vi "main.vi"() -> ()   [LabVIEW 2023, in "task_1.lvlib"]
doc: "A data monitoring system to to acquire and plot data."
uses:
  task_1.lvlib
  Controls/event_operations.ctl
  Controls/data_limits.ctl
  Controls/Queue_op.ctl
  <vilib>/Analysis/Matrix/Numeric/Conversions/Array To Matrix - RA.vi
  <vilib>/Analysis/Matrix/NI_Matrix.lvlib
panel:
  out "LED":bool
  out "error out":errorcluster
  in  "error in (no error)":errorcluster
  out "Temperature (°C):":dbl format="%#_4g"
  out "Current (mA):":dbl format="%#_4g"
  in  "Log Rate":dbl=1.0 min=1.0 step=1.0
  in  "Current. Low Limit mA":dbl min=0.0 max=100.0 format="%#.2g"
  in  "Current. High Limit mA":dbl=100.0 min=0.0 max=100.0 format="%#.2g"
  in  "Temp. Low Limit   °C":dbl min=0.0 max=100.0 format="%#.2g"
  in  "Temp. High Limit °C":dbl=100.0 min=0.0 max=100.0 format="%#.2g"
  in  "Exit":bool
  out "Chart":dbl[][](graph)=[[75.40776627883477, 3.2055013029279156]]
  in  "Start":bool
  # "Data Monitoring System"
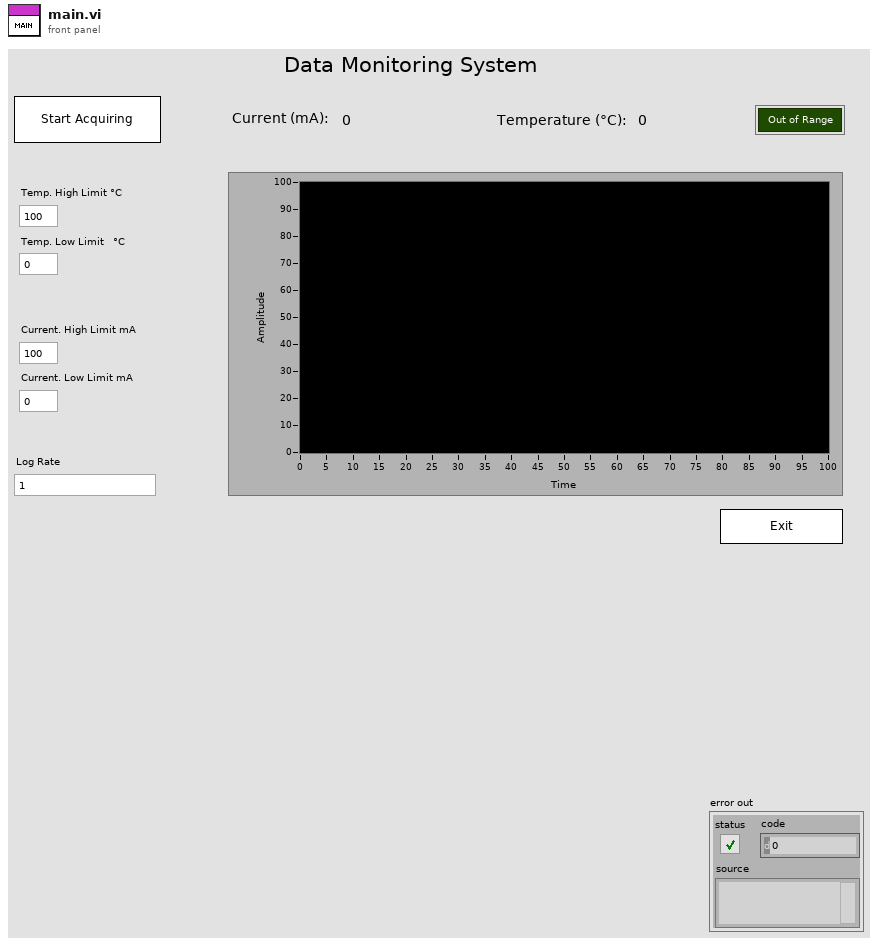
[diagram p1: front panel]
types:
  T1 = typedef "task_1.lvlib/data_limits.ctl" = cluster{"curr_h":dbl, "curr_l":dbl, "temp_h":dbl, "temp_l":dbl, "Acquiring?":bool}
  T2 = typedef "task_1.lvlib/event_operations.ctl" = enum16{"Create", "Generate", "Get_ref", "Destroy"}
  T3 = typedef "task_1.lvlib/Queue_op.ctl" = enum16{"Create", "Enqueue", "Dequeue", "Destroy"}
  T4 = enum32{"Invalid", "Standard", "Closed", "Hidden", "Minimized", "Maximized"}
  T5 = typedef "task_1.lvlib/Data_TC.ctl" = cluster{"Current":dbl, "Temperature":dbl}
  T6 = typedef "NI_Matrix.lvlib/RealMatrix.ctl" = dbl[][]
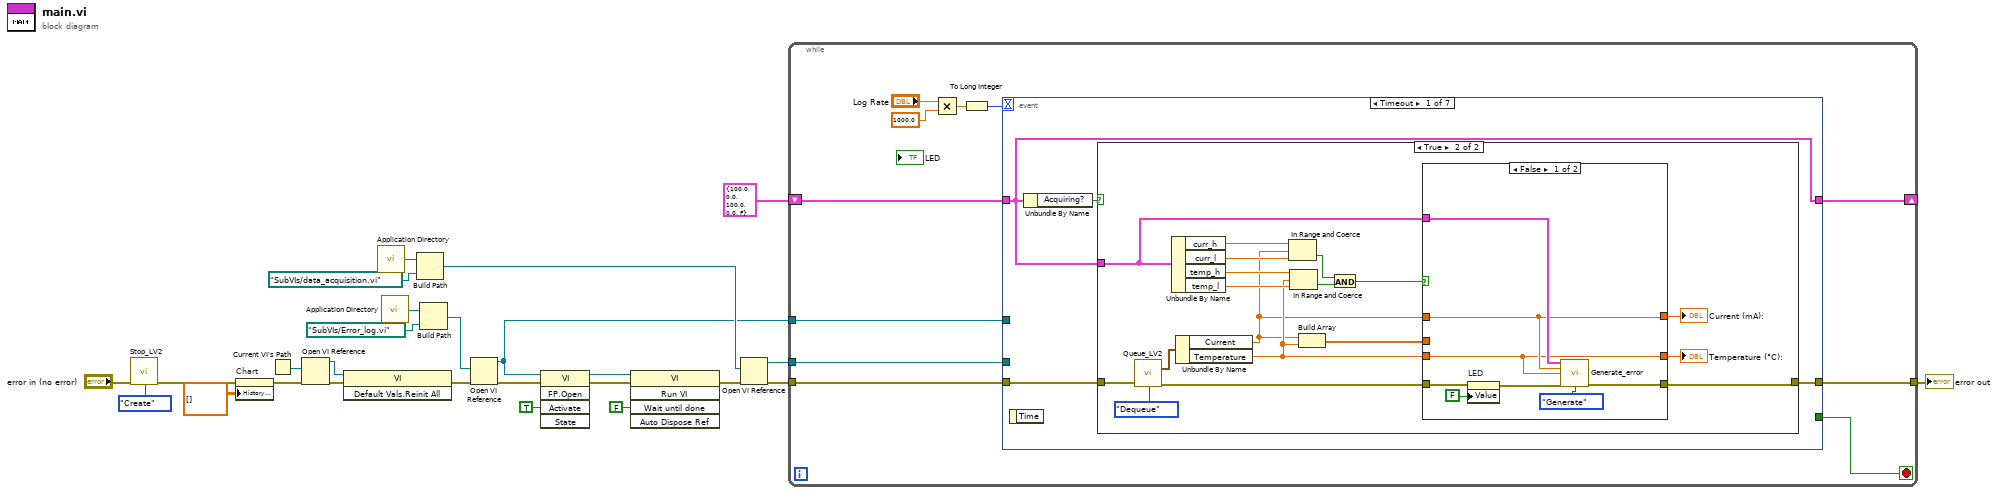
[diagram p0: block diagram]
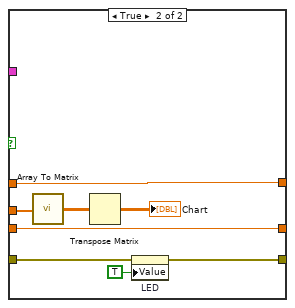
[diagram p3: hidden frame]
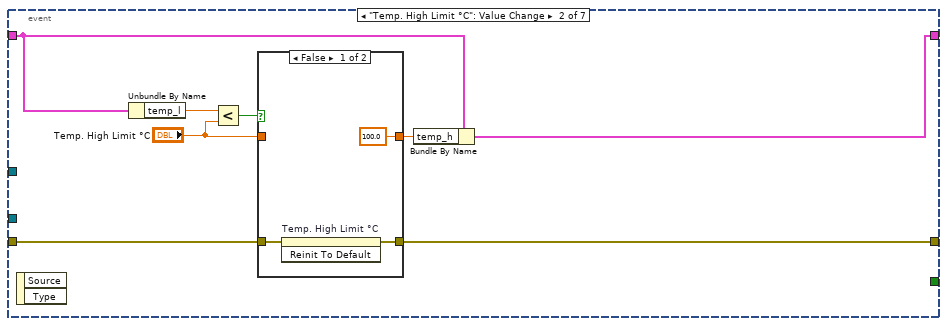
[diagram p4: hidden frame]
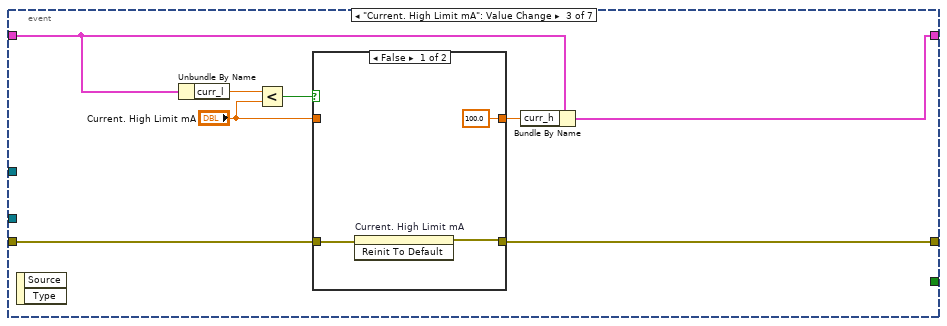
[diagram p6: hidden frame]
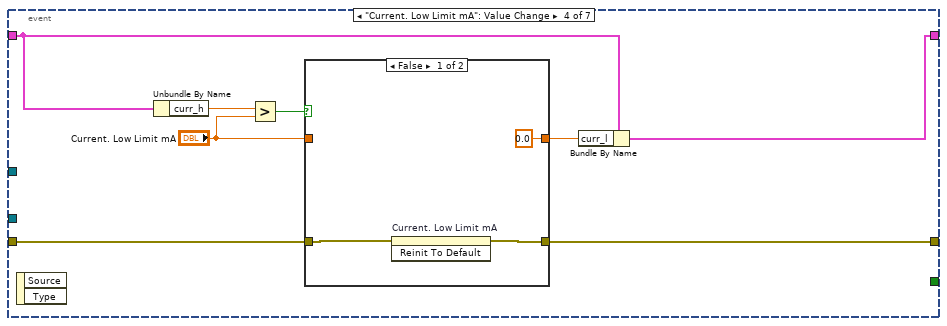
[diagram p8: hidden frame]
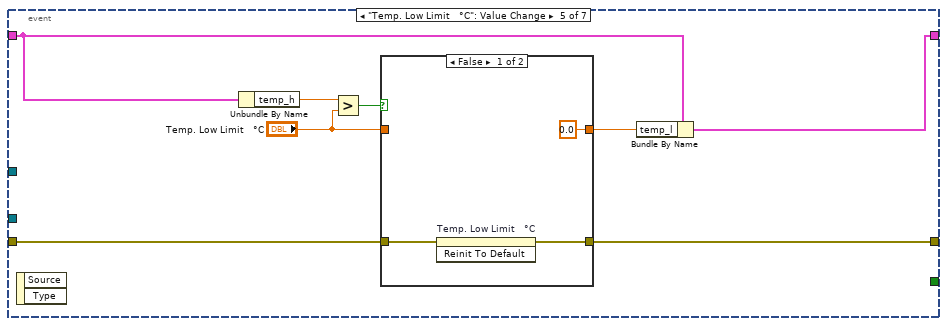
[diagram p10: hidden frame]
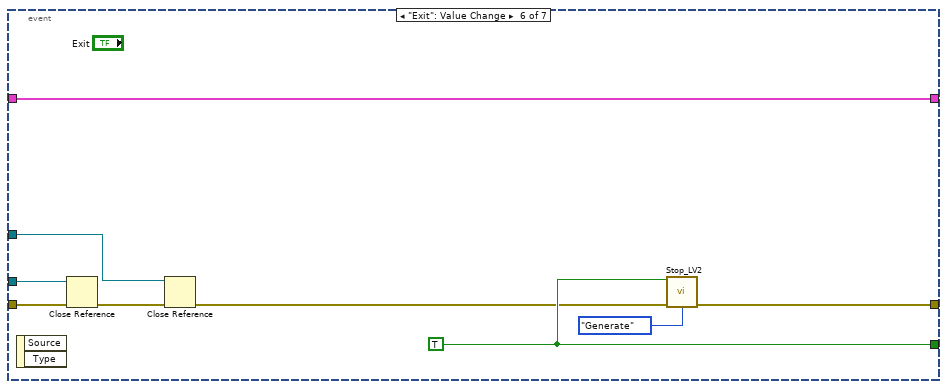
[diagram p12: hidden frame]
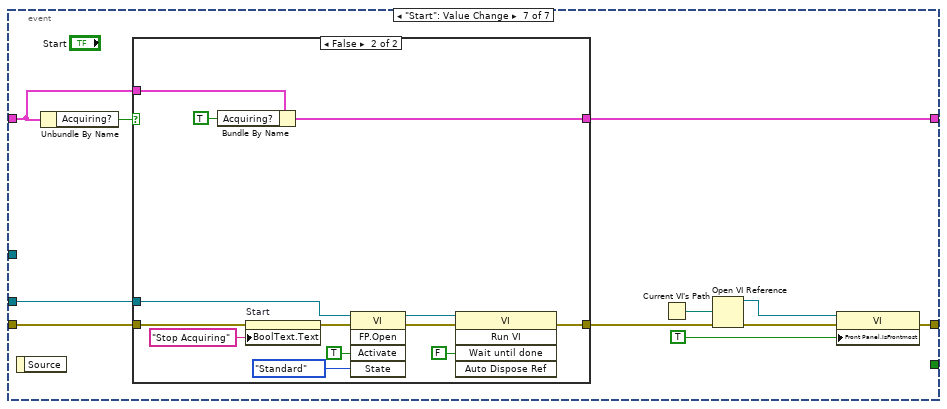
[diagram p13: hidden frame]
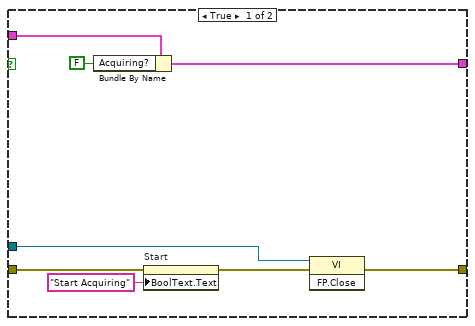
[diagram p14: hidden frame]
diagram:
  n1 = call "Stop_LV2.vi"("error in (no error)"="error in (no error)", "Operations"=event_operations."Create") -> ("error out"=w3:errorcluster)  [unwired: 12 in, 1 out]
  n2 = property on="Chart" class="WFChart (strict)"(error in=w3, "History Data"=dbl[][] []) -> (error out=w2:errorcluster)  [unwired: 1 in, 1 out]
  n3 = Current VI's Path() -> (path=w16:path)
  n4 = Open VI Reference(vi path=w16, error in (no error)=w2) -> (vi reference=w14:refnum<vi>, error out=w17:errorcluster)  [unwired: 4 in]
  n5 = invoke class="VI" method="Default Vals.Reinit All"(reference=w14, error in=w17) -> (error out=w15:errorcluster)  [unwired: 1 in, 2 out]
  n6 = call <vilib>:"Application Directory.vi"() -> ("Application Directory"=w26:path)
  n7 = call <vilib>:"Application Directory.vi"() -> ("Application Directory"=w11:path)
  n8 = Build Path(base path=w26, name or relative path=path "SubVIs/data_acquisition.vi") -> (appended path=w23:path)
  n9 = Build Path(base path=w11, name or relative path=path "SubVIs/Error_log.vi") -> (appended path=w10:path)
  n10 = Open VI Reference(vi path=w10, error in (no error)=w15) -> (vi reference=w4:refnum<vi>, error out=w13:errorcluster)  [unwired: 4 in]
  n11 = invoke class="VI" method="FP.Open"(reference=w4, error in=w13, "Activate"=TRUE ("Activate?")) -> (reference out=w7:refnum<vi>, error out=w8:errorcluster)  [unwired: 2 in, 3 out]
  n12 = invoke class="VI" method="Run VI"(reference=w7, error in=w8, "Wait until done"=FALSE ("Wait Until Done")) -> (error out=w9:errorcluster)  [unwired: 2 in, 4 out]
  n13 = Open VI Reference(vi path=w23, error in (no error)=w9) -> (vi reference=w22:refnum<vi>, error out=w24:errorcluster)  [unwired: 4 in]
  n14 = while {
    tunnel: w24 -> [w32]
    shift-right: [w31] -> _
    shift-left: T1 {"curr_h"=100.0, "curr_l"=0.0, "temp_h"=100.0, "temp_l"=0.0, "Acquiring?"=FALSE} ("Cluster") -> [w33]
    tunnel: [w30] -> w21
    tunnel: w22 -> [w29]
    tunnel: w4 -> [w27]
    stop <- w28 stop-if-true
    n15 = Multiply(x="Log Rate", y=1000.0) -> (x*y=w35:dbl)
    n16 = To Long Integer(number=w35) -> (32bit integer=w34:i32)
    n17 = event shown="[0] Timeout" {
      selector: _ -> [_ _ _ _ _ _ _]
      dyn-events: _ -> [_ _ _ _ _ _ _]
      timeout: w34 -> [_ _ _ _ _ _ _]
      tunnel: w33 -> [w38 w83 w96 w108 w122 w136 w146]
      tunnel: w32 -> [w40 w80 w93 w104 w117 w137 w147]
      tunnel: [w38 w84 w97 w105 w123 w136 w145] -> w31
      tunnel: [w39 w77 w92 w103 w116 w135 w141] -> w30
      tunnel: w29 -> [_ _ _ _ _ w132 w143]
      tunnel: [_ _ _ _ _ w133 _] -> w28
      tunnel: w27 -> [_ _ _ _ _ w129 _]
      event Timeout {
        n18 = event-data() -> ()  [unwired: 1 in, 1 out]
        n19 = Unbundle By Name(w38) -> ("Acquiring?"=w41:bool)
        n20 = case shown="True" w41 {
          tunnel: w40 -> [w42 w60]
          tunnel: [w42 w49] -> w39
          tunnel: w38 -> [_ w44]
          frame False {
          }
          frame True {
            n21 = call "Queue_LV2.vi"("error in (no error)"=w60, "Operation"=Queue_op."Dequeue") -> ("element out"=w59:T5, "error IO"=w50:errorcluster)  [unwired: 12 in]
            n22 = Unbundle By Name(w44) -> ("curr_h"=w58:dbl, "curr_l"=w57:dbl, "temp_h"=w56:dbl, "temp_l"=w55:dbl)
            n23 = Unbundle By Name(w59) -> ("Current"=w46:dbl, "Temperature"=w47:dbl)
            n24 = In Range and Coerce(upper limit=w58, x=w46, lower limit=w57) -> (In Range?=w52:bool)  [unwired: 1 out]
            n25 = In Range and Coerce(upper limit=w56, x=w47, lower limit=w55) -> (In Range?=w51:bool)  [unwired: 1 out]
            n26 = Build Array(w46, w47) -> (w53:dbl[])
            n27 = And(x=w52, y=w51) -> (x .and. y?=w54:bool)
            n28 = case shown="False" w54 {
              tunnel: w53 -> [_ w76]
              tunnel: w50 -> [w68 w73]
              tunnel: [w65 w72] -> w49
              tunnel: [w62 w70] -> w48
              tunnel: w47 -> [w62 w70]
              tunnel: w46 -> [w63 w69]
              tunnel: [w63 w69] -> w45
              tunnel: w44 -> [w64 _]
              frame False {
                n29 = property on="LED" class="Bool (strict)"(error in=w68, "Value"=FALSE ("LED")) -> (error out=w66:errorcluster)  [unwired: 1 in, 1 out]
                n30 = call "Generate_error.vi"("Data_in"=w64, "Current"=w63, "Temperature"=w62, "error in (no error)"=w66, "Operations"=event_operations."Generate") -> ("error IO"=w65:errorcluster)  [unwired: 9 in, 1 out]
              }
              frame True {
                n31 = call-poly <vilib>:"Array To Matrix.vi"("Real 1D Array"=w76) -> ("Real Matrix (Column Vector)"=w75:T6)
                n32 = Transpose Matrix(1:w75) -> (0:→"Chart":T6)
                n33 = property on="LED" class="Bool (strict)"(error in=w73, "Value"=TRUE ("LED")) -> (error out=w72:errorcluster)  [unwired: 1 in, 1 out]
              }
            }
            "Current (mA):" <- w45
            "Temperature (°C):" <- w48
          }
        }
      }
      event "Temp. High Limit °C": Value Change {
        n34 = event-data() -> ()  [unwired: 1 in, 2 out]
        n35 = Unbundle By Name(w83) -> ("temp_l"=w82:dbl)
        n36 = Less?(x=w82, y="Temp. High Limit °C") -> (x < y?=w81:bool)
        n37 = case shown="False" w81 {
          tunnel: w80 -> [w86 w88]
          tunnel: "Temp. High Limit °C" -> [_ w89]
          tunnel: [100.0 ("Temp. High Limit °C") w89] -> w78
          tunnel: [w85 w88] -> w77
          frame False {
            n38 = invoke on="Temp. High Limit °C" class="DigNum (strict)" method="Reinit To Default"(error in=w86) -> (error out=w85:errorcluster)  [unwired: 2 in, 2 out]
          }
          frame True {
          }
        }
        n39 = Bundle By Name(cluster=w83, "temp_h"=w78) -> (w84:T1)
      }
      event "Current. High Limit mA": Value Change {
        n40 = event-data() -> ()  [unwired: 1 in, 2 out]
        n41 = Unbundle By Name(w96) -> ("curr_l"=w95:dbl)
        n42 = Less?(x=w95, y="Current. High Limit mA") -> (x < y?=w94:bool)
        n43 = case shown="False" w94 {
          tunnel: w93 -> [w100 w102]
          tunnel: [w99 w102] -> w92
          tunnel: "Current. High Limit mA" -> [_ w101]
          tunnel: [100.0 ("Current. High Limit mA") w101] -> w90
          frame False {
            n44 = invoke on="Current. High Limit mA" class="DigNum (strict)" method="Reinit To Default"(error in=w100) -> (error out=w99:errorcluster)  [unwired: 2 in, 2 out]
          }
          frame True {
          }
        }
        n45 = Bundle By Name(cluster=w96, "curr_h"=w90) -> (w97:T1)
      }
      event "Current. Low Limit mA": Value Change {
        n46 = event-data() -> ()  [unwired: 1 in, 2 out]
        n47 = Unbundle By Name(w108) -> ("curr_h"=w110:dbl)
        n48 = Greater?(x=w110, y="Current. Low Limit mA") -> (0:w109:bool)
        n49 = case shown="False" w109 {
          tunnel: "Current. Low Limit mA" -> [_ w115]
          tunnel: [0.0 ("Current. Low Limit mA") w115] -> w106
          tunnel: w104 -> [w113 w114]
          tunnel: [w112 w114] -> w103
          frame False {
            n50 = invoke on="Current. Low Limit mA" class="DigNum (strict)" method="Reinit To Default"(error in=w113) -> (error out=w112:errorcluster)  [unwired: 2 in, 2 out]
          }
          frame True {
          }
        }
        n51 = Bundle By Name(cluster=w108, "curr_l"=w106) -> (w105:T1)
      }
      event "Temp. Low Limit   °C": Value Change {
        n52 = event-data() -> ()  [unwired: 1 in, 2 out]
        n53 = Unbundle By Name(w122) -> ("temp_h"=w121:dbl)
        n54 = Greater?(x=w121, y="Temp. Low Limit   °C") -> (0:w120:bool)
        n55 = case shown="False" w120 {
          tunnel: "Temp. Low Limit   °C" -> [_ w128]
          tunnel: [0.0 ("Temp. Low Limit   °C") w128] -> w118
          tunnel: w117 -> [w125 w127]
          tunnel: [w124 w127] -> w116
          frame False {
            n56 = invoke on="Temp. Low Limit   °C" class="DigNum (strict)" method="Reinit To Default"(error in=w125) -> (error out=w124:errorcluster)  [unwired: 2 in, 2 out]
          }
          frame True {
          }
        }
        n57 = Bundle By Name(cluster=w122, "temp_l"=w118) -> (w123:T1)
      }
      event "Exit": Value Change {
        w133 = TRUE
        n58 = event-data() -> ()  [unwired: 1 in, 2 out]
        n59 = Close Reference(reference=w132, error in (no error)=w137) -> (error out=w131:errorcluster)
        n60 = Close Reference(reference=w129, error in (no error)=w131) -> (error out=w130:errorcluster)
        n61 = call "Stop_LV2.vi"("Stop"=w133, "error in (no error)"=w130, "Operations"=event_operations."Generate") -> ("error out"=w135:errorcluster)  [unwired: 11 in, 1 out]
      }
      event "Start": Value Change {
        n62 = event-data() -> ()  [unwired: 1 in, 1 out]
        n63 = Unbundle By Name(w146) -> ("Acquiring?"=w148:bool)
        n64 = case shown="False" w148 {
          tunnel: w147 -> [w156 w169]
          tunnel: w146 -> [w154 w167]
          tunnel: [w152 w165] -> w145
          tunnel: [w150 w161] -> w144
          tunnel: w143 -> [w149 w162]
          frame True {
            n65 = Bundle By Name(cluster=w154, "Acquiring?"=FALSE) -> (w152:T1)
            n66 = property on="Start" class="Bool"(error in=w156, "BoolText.Text"="Start Acquiring" ("Boolean Text.Text")) -> (error out=w151:errorcluster)  [unwired: 1 in, 1 out]
            n67 = invoke class="VI" method="FP.Close"(reference=w149, error in=w151) -> (error out=w150:errorcluster)  [unwired: 1 in, 2 out]
          }
          frame False {
            n68 = Bundle By Name(cluster=w167, "Acquiring?"=TRUE) -> (w165:T1)
            n69 = property on="Start" class="Bool"(error in=w169, "BoolText.Text"="Stop Acquiring" ("Boolean Text.Text")) -> (error out=w164:errorcluster)  [unwired: 1 in, 1 out]
            n70 = invoke class="VI" method="FP.Open"(reference=w162, error in=w164, "Activate"=TRUE ("Activate?"), "State"=T4."Standard") -> (reference out=w160:refnum<vi>, error out=w163:errorcluster)  [unwired: 1 in, 3 out]
            n71 = invoke class="VI" method="Run VI"(reference=w160, error in=w163, "Wait until done"=FALSE ("Wait Until Done")) -> (error out=w161:errorcluster)  [unwired: 2 in, 4 out]
          }
        }
        n72 = Current VI's Path() -> (path=w138:path)
        n73 = Open VI Reference(vi path=w138, error in (no error)=w144) -> (vi reference=w140:refnum<vi>, error out=w142:errorcluster)  [unwired: 4 in]
        n74 = property class="VI"(reference=w140, error in=w142, "Front Panel.IsFrontmost"=TRUE ("Front Panel Window:Is Frontmost")) -> (error out=w141:errorcluster)  [unwired: 1 out]
      }
    }
  }
  "error out" <- w21
